vi "InitTankPDE.vi"(7 "water_level":dbl, 8 "error in (no error)":errorcluster, 9 "a":dbl, 10 "k":dbl=1.0, 11 "tank_resolution":T1) -> (0 "error out":errorcluster, 3 "PDE out":refnum<class "NI_PDE.lvclass">)   [LabVIEW 2020]
uses:
  <vilib>/gmath/pde.llb/PDEClass/NI_PDE.lvclass
  TankResolution.ctl
  TimeSteps.ctl
  XSteps.ctl
  YSteps.ctl
  <vilib>/gmath/pde.llb/Define 2D Heat PDE (Numeric).vi
  <vilib>/gmath/pde.llb/Define 2D Heat PDE Domain (Rect).vi
  <vilib>/gmath/NI_PDE.lvlib
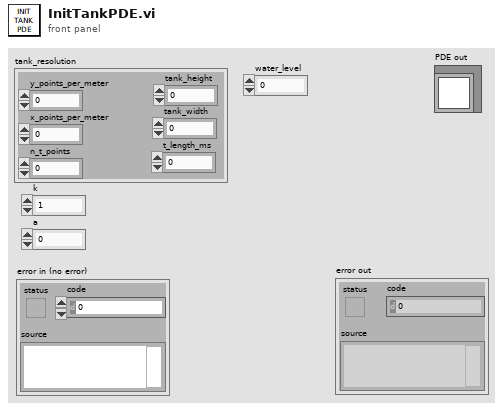
[diagram p1: front panel]
types:
  T1 = typedef "TankResolution.ctl" = cluster{"y_points_per_meter":i32, "x_points_per_meter":i32, "n_t_points":i32, "tank_height":dbl, "tank_width":dbl, "t_length_ms":u32}
  T2 = typedef "YSteps.ctl" = cluster{"start y":dbl, "end y":dbl, "# of y-points":i32}
  T3 = typedef "XSteps.ctl" = cluster{"start x":dbl, "end x":dbl, "# of x-points":i32}
  T4 = typedef "TimeSteps.ctl" = cluster{"initial t":dbl, "final t":dbl, "# of t-points":i32}
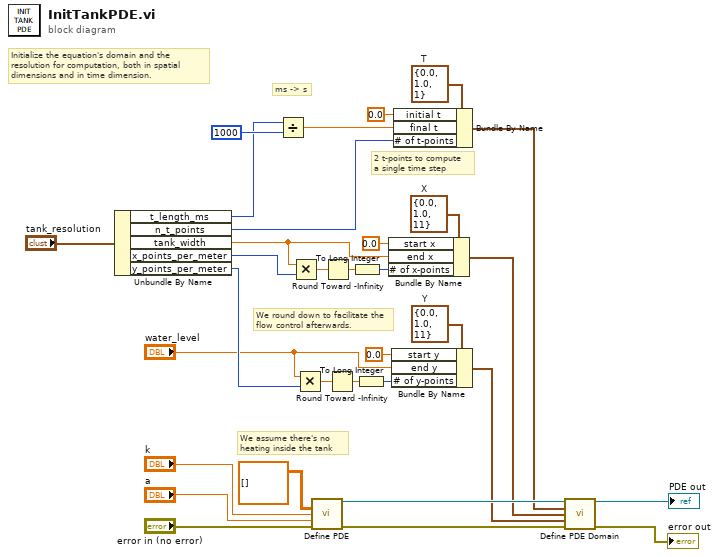
[diagram p0: block diagram]
diagram:
  w24 = T2 {"start y"=0.0, "end y"=1.0, "# of y-points"=11}  # Y
  w27 = T3 {"start x"=0.0, "end x"=1.0, "# of x-points"=11}  # X
  w30 = T4 {"initial t"=0.0, "final t"=1.0, "# of t-points"=1}  # T
  # "We round down to facilitate the flow control afterwards."
  # "Initialize the equation's domain and the resolution for computation, both in spatial dimensions and in time dimension."
  # "ms -> s"
  # "2 t-points to compute\na single time step"
  # "We assume there's no\nheating inside the tank"
  n1 = Unbundle By Name("tank_resolution") -> ("t_length_ms"=w13:u32, "n_t_points"=w2:i32, "tank_width"=w11:dbl, "x_points_per_meter"=w12:i32, "y_points_per_meter"=w4:i32)
  n2 = Divide(x=w13, y=u32 1000 ("x")) -> (x/y=w1:dbl)
  n3 = Multiply(x=w11, y=w12) -> (x*y=w10:dbl)
  n4 = Multiply(x="water_level", y=w4) -> (x*y=w7:dbl)
  n5 = call-poly <vilib>:"Define PDE.vi"("F(t, x, y)"=dbl[][][] [], "k"="k", "a"="a", "error in (no error)"="error in (no error)") -> ("PDE out"=w31:refnum<class "NI_PDE.lvclass">, "error out"=w21:errorcluster)  [unwired: 10 in]
  n6 = Round Toward -Infinity(1:w10) -> (0:w9:dbl)
  n7 = Round Toward -Infinity(1:w7) -> (0:w6:dbl)
  n8 = To Long Integer(number=w9) -> (32bit integer=w8:i32)
  n9 = To Long Integer(number=w6) -> (32bit integer=w5:i32)
  n10 = Bundle By Name(cluster=w27, "start x"=0.0, "end x"=w11, "# of x-points"=w8) -> (w25:T3)
  n11 = Bundle By Name(cluster=w24, "start y"=0.0, "end y"="water_level", "# of y-points"=w5) -> (w22:T2)
  n12 = Bundle By Name(cluster=w30, "initial t"=0.0, "final t"=w1, "# of t-points"=w2) -> (w28:T4)
  n13 = call-poly <vilib>:"Define PDE Domain.vi"("PDE in"=w31, "T"=w28, "X"=w25, "Y"=w22, "error in (no error)"=w21) -> ("PDE out"=→"PDE out":refnum<class "NI_PDE.lvclass">, "error out"=→"error out":errorcluster)  [unwired: 9 in]
